vi "Read Reference.vi"(0 "Wave File":path, 7 "refUnits":string="refSPL", 11 "error in (no error)":errorcluster) -> (4 "Reference (dB)":dbl, 8 "Units":string, 15 "error out":errorcluster)   [LabVIEW 2020, in "File.lvclass"]
uses:
  File.lvclass
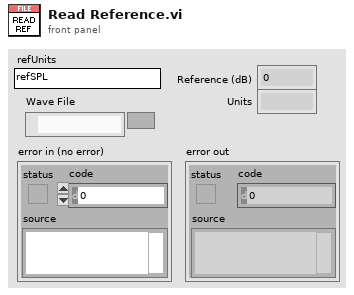
[diagram p1: front panel]
types:
  T1 = typedef "Wave-EPL Chunk Variable.ctl" = cluster{"Name":string, "Value":dbl}
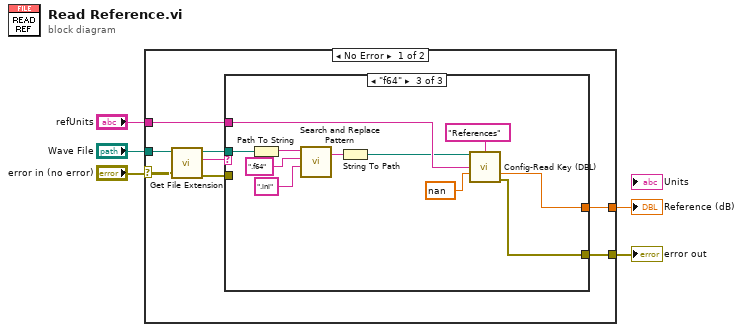
[diagram p0: block diagram]
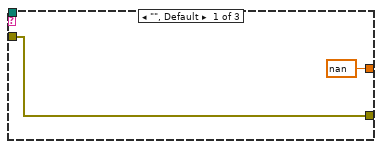
[diagram p2: hidden frame]
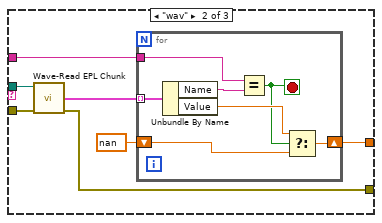
[diagram p3: hidden frame]
diagram:
  n1 = case shown="No Error" "error in (no error)" {
    selector: "error in (no error)" -> [w7 w41]
    tunnel: [w13 w41] -> w4
    tunnel: "Wave File" -> [w8 _]
    tunnel: [w12 _] -> w2
    tunnel: "refUnits" -> [w11 _]
    frame No Error {
      n2 = call <vilib>:"Get File Extension.vi"("error in (no error)"=w7, "file"=w8) -> ("error out"=w10:errorcluster, "lowercase file extension"=w6:string, "dup file"=w9:path)  [unwired: 5 in, 2 out]
      n3 = case shown="\"f64\"" w6 {
        tunnel: [w15 w20 w36] -> w13
        tunnel: [nan w19 w38] -> w12
        tunnel: w11 -> [_ w18 w39]
        tunnel: w10 -> [w15 w17 _]
        tunnel: w9 -> [_ w16 w35]
        frame "", Default {
        }
        frame "wav" {
          n4 = call "Wave-Read EPL Chunk.vi"("Wave File"=w16, "error in (no error)"=w17) -> ("EPL Variables"=w22:T1[], "error out"=w20:errorcluster)  [unwired: 12 in]
          n5 = for {
            tunnel: w22 -> [w29] mode=indexing
            shift-right: [w25] -> w19
            shift-left: nan -> [w26]
            tunnel: w18 -> [w23]
            stop <- w24 stop-if-true
            n6 = Unbundle By Name(w29) -> ("Name"=w28:string, "Value"=w27:dbl)
            n7 = Equal?(x=w23, y=w28) -> (x = y?=w24:bool)
            n8 = Select(t=w27, s=w24, f=w26) -> (s? t:f=w25:dbl)
          }
        }
        frame "f64" {
          n9 = Path To String(path=w35) -> (string=w34:string)
          n10 = call <vilib>:"Search and Replace Pattern.vi"("string"=w34, "regular expression (\"\")"=".f64" ("regular expression (\"\")"), "replace string (\"\")"=".ini" ("replace string (\"\")")) -> ("result string"=w31:string)  [unwired: 2 in, 1 out]
          n11 = String To Path(string=w31) -> (path=w30:path)
          n12 = call "Config-Read Key (DBL).vi"("configuration file path"=w30, "section"="References", "key"=w39, "default"=nan) -> ("value"=w38:dbl, "error out"=w36:errorcluster)  [unwired: 8 in, 2 out]
        }
      }
    }
    frame Error {
    }
  }
  "error out" <- w4
  "Reference (dB)" <- w2
